vi "createNewPage.vi"(6 "Set as active (T)":bool=TRUE, 8 "error in (no error)":errorcluster, 10 "Page Name":string, 11 "MS-Word in":refnum<class "MS-Word.lvclass">) -> (0 "error out":errorcluster, 1 "Created?":bool, 2 "Created Page Name":string, 3 "MS-Word out":refnum<class "MS-Word.lvclass">)   [LabVIEW 2017, in "LabVIEW NPOI.lvlib" / "MS-Word.lvclass"]
uses:
  MS-Word.lvclass
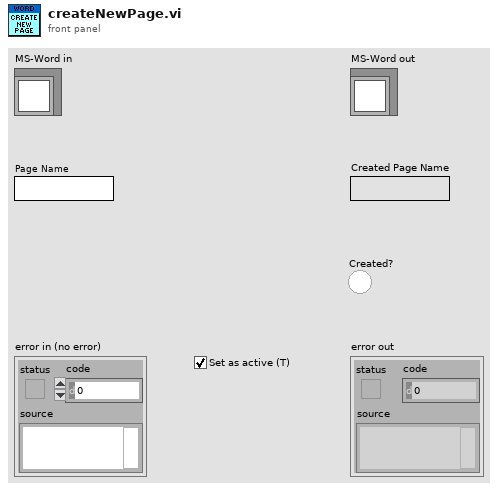
[diagram p1: front panel]
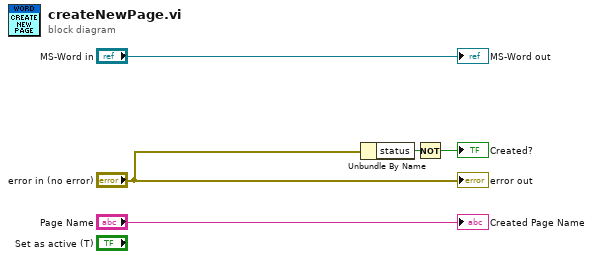
[diagram p0: block diagram]
diagram:
  n1 = Unbundle By Name("error in (no error)") -> ("status"=w3:bool)
  n2 = Not(x=w3) -> (.not. x?=→"Created?":bool)
  "error out" <- "error in (no error)"
  "MS-Word out" <- "MS-Word in"
  "Created Page Name" <- "Page Name"
